vi "Read and Save as TDMS.vi"   [LabVIEW 2020, in "Agilent 90000 Series.lvlib"]
doc: "Returns scaled/unscaled data points from the instrument and save them into a TDMS file on the specified format."
uses:
  Agilent 90000 Series.lvlib
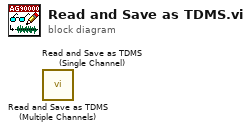
[diagram p0: block diagram]
diagram:
  n1 = call "Read and Save as TDMS (Multiple Channels).vi"() -> ()  [unwired: 12 in, 4 out]
  n2 = call "Read and Save as TDMS (Single Channel).vi"() -> ()  [unwired: 12 in, 4 out]
